vi "KE622x -- Get Trig Layer Params.vi"(0 "Resource In":refnum<visa-resource-name>, 1 "Check For SCPI Errors? (T)":bool=TRUE, 11 "error in (no error)":errorcluster) -> (4 "Resource Out (dupl)":refnum<visa-resource-name>, 8 "Trig Layer Params":T1, 15 "error out":errorcluster)   [LabVIEW 2018, in "Keithley 622x.lvlib"]
doc: "Returns the parameters for the 'Trigger' layer of the trigger model."
uses:
  Keithley 622x.lvlib
  Low Level/Typedefs/KE622x -- Trig Source.ctl
  Low Level/Typedefs/KE622x -- Trig Link Line.ctl
  Low Level/Typedefs/KE622x -- Trig Output Mode.ctl
  Typedefs/KE622x -- Trig Layer Params.ctl
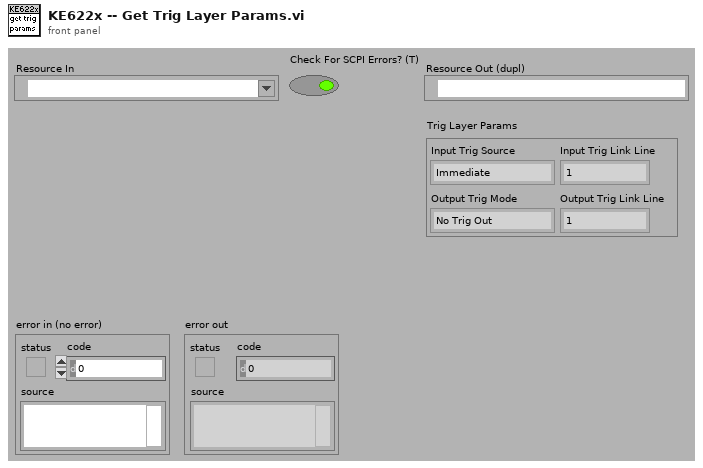
[diagram p1: front panel]
types:
  T1 = typedef "Keithley 622x.lvlib/KE622x -- Trig Layer Params.ctl" = cluster{"Input Trig Source":T2, "Input Trig Link Line":T3, "Output Trig Mode":T4, "Output Trig Link Line":T3}
  T2 = typedef "Keithley 622x.lvlib/KE622x -- Trig Source.ctl" = enum16{"Immediate", "Trigger Link"}
  T3 = typedef "Keithley 622x.lvlib/KE622x -- Trig Link Line.ctl" = enum16{"1", "2", "3", "4", "5", "6"}
  T4 = typedef "Keithley 622x.lvlib/KE622x -- Trig Output Mode.ctl" = enum16{"No Trig Out", "Source Turn On", "After Source Delay"}
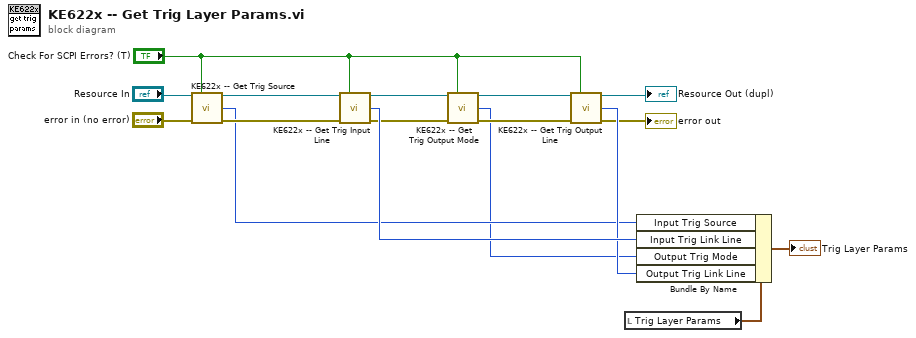
[diagram p0: block diagram]
diagram:
  n1 = call "KE622x -- Get Trig Source.vi"("Resource In"="Resource In", "Check For SCPI Errors? (T)"="Check For SCPI Errors? (T)", "error in (no error)"="error in (no error)") -> ("Resource Out (dupl)"=w7:refnum<visa-resource-name>, "Trig Source"=w3:T2, "error out"=w6:errorcluster)  [unwired: 10 in]
  n2 = call "KE622x -- Get Trig Input Line.vi"("Resource In"=w7, "Check For SCPI Errors? (T)"="Check For SCPI Errors? (T)", "error in (no error)"=w6) -> ("Resource Out (dupl)"=w5:refnum<visa-resource-name>, "Trig Input Line"=w11:T3, "error out"=w4:errorcluster)  [unwired: 10 in]
  n3 = call "KE622x -- Get Trig Output Mode.vi"("Resource In"=w5, "Check For SCPI Errors? (T)"="Check For SCPI Errors? (T)", "error in (no error)"=w4) -> ("Resource Out (dupl)"=w14:refnum<visa-resource-name>, "Trig Output Mode"=w2:T4, "error out"=w15:errorcluster)  [unwired: 10 in]
  n4 = call "KE622x -- Get Trig Output Line.vi"("Resource In"=w14, "Check For SCPI Errors? (T)"="Check For SCPI Errors? (T)", "error in (no error)"=w15) -> ("Resource Out (dupl)"=→"Resource Out (dupl)":refnum<visa-resource-name>, "Trig Output Line"=w10:T3, "error out"=→"error out":errorcluster)  [unwired: 10 in]
  n5 = local read "Trig Layer Params"() -> (w12:T1)
  n6 = Bundle By Name(cluster=w12, "Input Trig Source"=w3, "Input Trig Link Line"=w11, "Output Trig Mode"=w2, "Output Trig Link Line"=w10) -> (→"Trig Layer Params":T1)
